vi "LVClass_WavefrontCorrector Check Relative Position.vi"(0 "WavefrontCorrector in":refnum<class "WavefrontCorrector.lvclass">, 5 "Relative Positions":T1, 11 "error in (no error)":errorcluster) -> (4 "WavefrontCorrector out":refnum<class "WavefrontCorrector.lvclass">, 6 "Relative Positions OUT":T1, 15 "error out":errorcluster)   [LabVIEW 2020, in "WavefrontCorrector.lvclass"]
doc: "Assert if requested relative positions satisfy current preferences.\n\n--------------------------------------------------------------------------------\n\n<B>correctorIn </B> : WavefrontCorrector object.\n<B>correctorOut </B> : WavefrontCorrector object.\n<B>position </B> : Requested relatives positions.\n<B>ErrorIn </B> : Error\n<B>ErrorOut </B> : Error\n\n--------------------------------------------------------------------------------"
uses:
  WavefrontCorrector.lvclass
  Controls/Wavefront Corrector Position.ctl
  WavefrontCorrector.lvclass/WavefrontCorrector.ctl
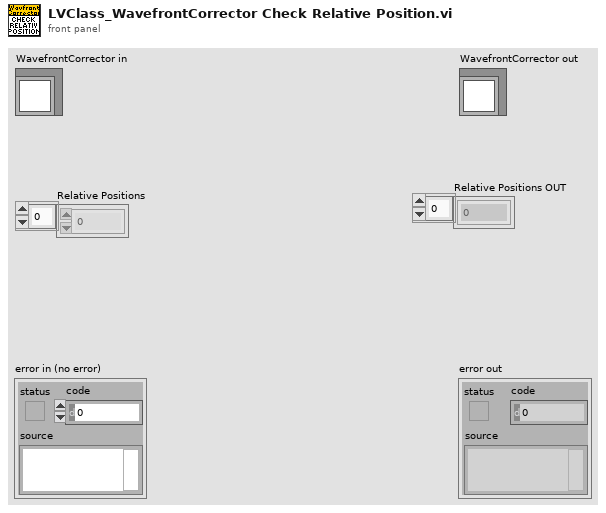
[diagram p1: front panel]
types:
  T1 = typedef "Wavefront Corrector Position.ctl" = sgl[]
  T2 = typedef "ClassID.ctl" = i64
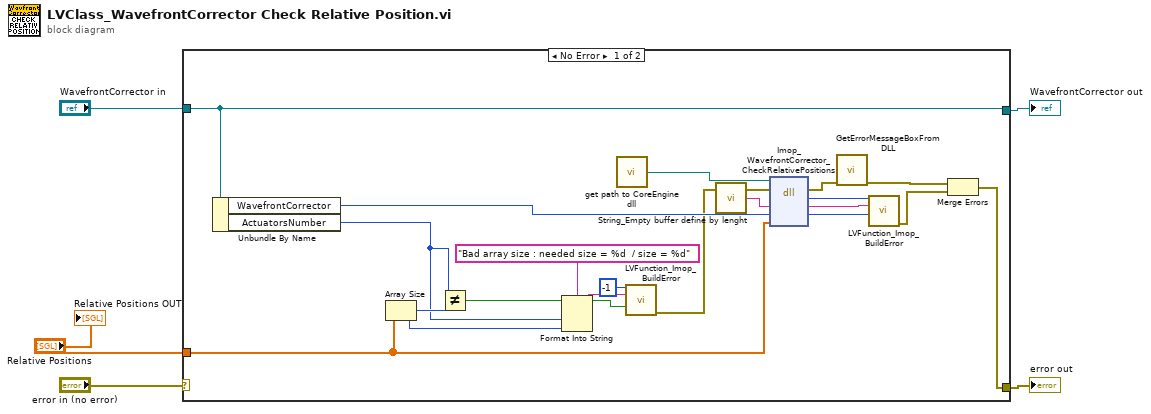
[diagram p0: block diagram]
diagram:
  n1 = case shown="No Error" "error in (no error)" {
    selector: "error in (no error)" -> [_ w26]
    tunnel: [w16 w26] -> w2
    tunnel: [w15 w25] -> w3
    tunnel: "WavefrontCorrector in" -> [w15 w25]
    tunnel: "Relative Positions" -> [w7 _]
    frame No Error {
      n2 = Unbundle By Name(w15) -> ("WavefrontCorrector"=w17:T2, "ActuatorsNumber"=w9:i32)
      n3 = Array Size(array=w7) -> (size(s)=w12:i32)
      n4 = Not Equal?(x=w9, y=w12) -> (x != y?=w11:bool)
      n5 = Format Into String(format string="Bad array size : needed size = %d  / size = %d" ("String to Prepend to source (\"\")"), w9, w12) -> (resulting string=w13:string)  [unwired: 2 in, 1 out]
      n6 = call "get path to CoreEngine dll.vi"() -> ("path to wavekit library"=w21:path)  [unwired: 14 in, 1 out]
      n7 = call "LVFunction_Imop_BuildError.vi"("code"=-1, "String to Prepend to source (\"\")"=w13, "Activate error? (true)"=w11) -> ("error out"=w8:errorcluster)  [unwired: 12 in]
      n8 = call "String_Empty buffer define by lenght.vi"() -> ("Empty buffer"=w22:string)  [unwired: 1 in]
      n9 = dll-call lib="D:/soft/HASO_v3/SVN_trunk/ImOpCoreEngine4_LV2011/DLLs/c_interface_vc100.dll" fn="Imop_WavefrontCorrector_CheckRelativePositions"(path in=w21, error in=w8, "message"=w22, "WavefrontCorrection"=w17, "Relative Position"=w7) -> (error out=w20:errorcluster, "return type"=w24:i32, "message"=w23:string, "WavefrontCorrection"=w6:i64)  [unwired: 2 in, 1 out]
      n10 = call "GetErrorMessageBoxFromDLL.vi"("error IN"=w20) -> ("error OUT"=w19:errorcluster)  [unwired: 10 in]
      n11 = call "LVFunction_Imop_BuildError.vi"("code"=w24, "String to Prepend to source (\"\")"=w23, "Adresse"=w6) -> ("error out"=w18:errorcluster)  [unwired: 12 in]
      n12 = Merge Errors(w19, w18) -> (w16:errorcluster)
    }
    frame Error {
    }
  }
  "error out" <- w2
  "WavefrontCorrector out" <- w3
  "Relative Positions OUT" <- "Relative Positions"
